vi "Type Mismatch.vi"(7 "caller name":string, 8 "error in (no error)":errorcluster, 9 "Data Type Requested":T1, 10 "True Type":T1, 11 "Tag":string) -> (0 "error out":errorcluster)   [LabVIEW 2021, in "CVT.lvlib" / "Current Value Table.lvlib"]
doc: "This VI throws an error if the specified types do not match."
uses:
  Current Value Table.lvlib
  Type Defs/Data Types.ctl
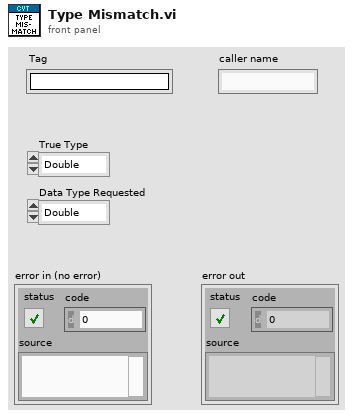
[diagram p1: front panel]
types:
  T1 = typedef "CVT.lvlib/Current Value Table.lvlib/Data Types.ctl" = enum16{"Double", "Single", "I64", "I32", "I16", "I8", "U64", "U32", "U16", "U8", "String", "Boolean", "Array of U8", "Array of U16", "Array of U32", "Array of U64", "Array of I64", "Array of I32", "Array of I16", "Array of I8", "Array of Double", "Array of Single", "Array of Boolean", "Array of String"}
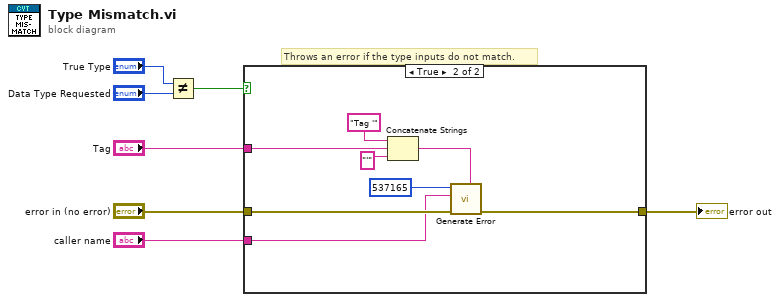
[diagram p0: block diagram]
diagram:
  # "Throws an error if the type inputs do not match."
  n1 = Not Equal?(x="True Type", y="Data Type Requested") -> (x != y?=w6:bool)
  n2 = case shown="True" w6 {
    tunnel: [w8 w10] -> w7
    tunnel: "Tag" -> [_ w16]
    tunnel: "error in (no error)" -> [w8 w11]
    tunnel: "caller name" -> [_ w9]
    frame False {
    }
    frame True {
      n3 = Concatenate Strings("Tag '" ("string"), w16, "'" ("string")) -> (w13:string)
      n4 = call "Generate Error.vi"("<append> (\"\")"=w13, "error in"=w11, "caller name"=w9, "code"=537165) -> ("error out"=w10:errorcluster)  [unwired: 7 in]
    }
  }
  "error out" <- w7
